vi "Write IConfigure.vi"(8 "error in (no error)":errorcluster, 10 "IConfigure":refnum<class "IConfigure.lvclass">, 11 "Camera Base in":refnum<class "Camera Base.lvclass">) -> (0 "error out":errorcluster, 3 "Camera Base out":refnum<class "Camera Base.lvclass">)   [LabVIEW 2023, in "HAL.lvlib" / "Camera Base.lvclass"]
uses:
  Camera Base.lvclass
  Camera Base.lvclass/Camera Base.ctl
  Interfaces/IConfigure/IConfigure.lvclass
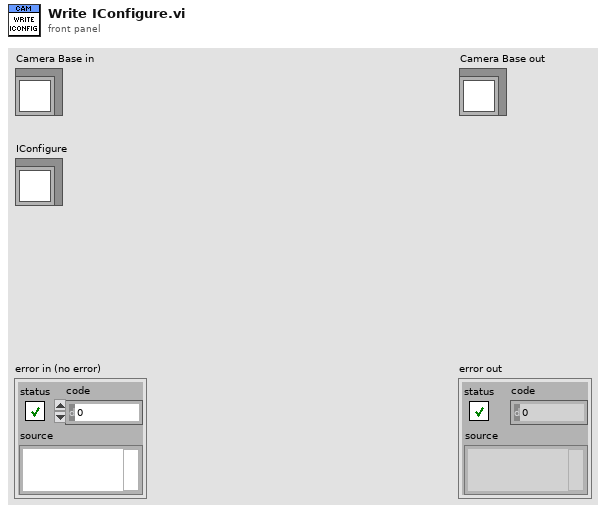
[diagram p1: front panel]
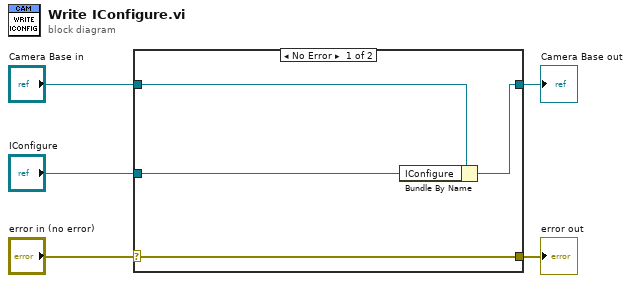
[diagram p0: block diagram]
diagram:
  n1 = case shown="No Error" "error in (no error)" {
    selector: "error in (no error)" -> [w9 w10]
    tunnel: [w9 w10] -> w4
    tunnel: [w7 w11] -> w2
    tunnel: "Camera Base in" -> [w8 w11]
    tunnel: "IConfigure" -> [w6 _]
    frame No Error {
      n2 = Bundle By Name(cluster=w8, "IConfigure"=w6) -> (w7:refnum<class "Camera Base.lvclass">)
    }
    frame Error {
    }
  }
  "error out" <- w4
  "Camera Base out" <- w2
